vi "Calibrate.vi"() -> ()   [LabVIEW 2017]
uses:
  <vilib>/myRIO/Instrument Drivers/Onboard IO/AI/vis/Read.vi
  <vilib>/myRIO/Instrument Drivers/Onboard IO/AI/vis/Smart Open.vi
  <vilib>/Utility/error.llb/Error Cluster From Error Code.vi
  <vilib>/myRIO/Common/Instrument Driver Framework/myRIO v1.0/AI/vis/myRIO v1.0 Read AI.vi
panel:
  in  "Sampling rate(Hz)":dbl
  out "Theta":dbl
  in  "t offset":dbl
  in  "t amp":dbl=1.0
  out "Position":dbl
  in  "x offset":dbl
  in  "x amp":dbl=1.0
  out "Theta voltage":dbl
  out "X voltage":dbl
  in  "Stop Button":bool
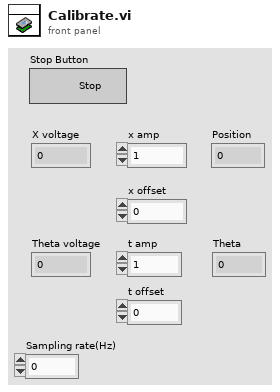
[diagram p1: front panel]
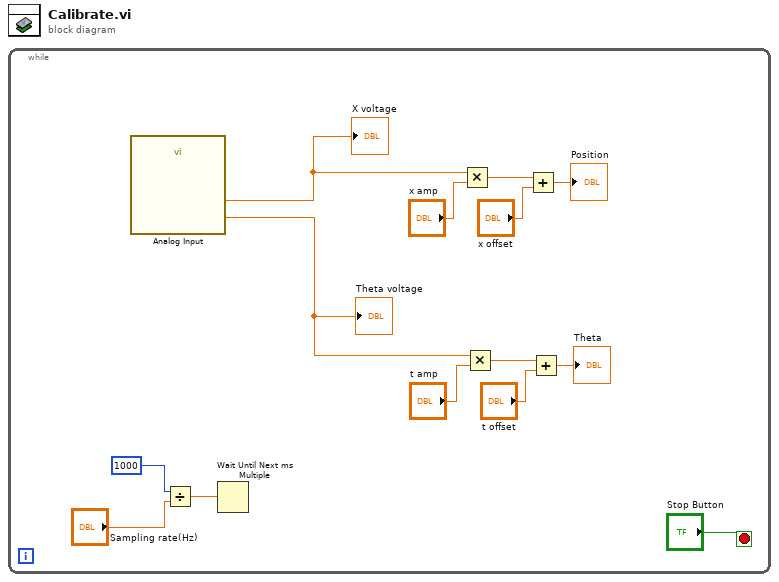
[diagram p0: block diagram]
diagram:
  n1 = while {
    stop <- "Stop Button" stop-if-true
    n2 = call "Analog Input"() -> ("C/AI0"=w5:dbl, "C/AI1"=w4:dbl)  [unwired: 25 in, 1 out]
    "X voltage" <- w5
    "Theta voltage" <- w4
    n3 = Divide(x=1000, y="Sampling rate(Hz)") -> (x/y=w1:dbl)
    n4 = Wait Until Next ms Multiple(millisecond multiple=w1) -> ()  [unwired: 1 out]
    n5 = Multiply(x=w5, y="x amp") -> (x*y=w13:dbl)
    n6 = Multiply(x=w4, y="t amp") -> (x*y=w9:dbl)
    n7 = Add(x=w13, y="x offset") -> (x+y=→"Position":dbl)
    n8 = Add(x=w9, y="t offset") -> (x+y=→"Theta":dbl)
  }
